vi "DG535.set internal trigger rate.vi"(0 "i ref in":refnum<vi>, 7 "internal trigger rate":dbl=0.001 min=0.001 max=1000000.0 format="%.3f", 11 "error in (no error)":errorcluster) -> (4 "i ref out":refnum<vi>, 15 "error out":errorcluster)   [LabVIEW 2014, in "DG535.lvlib"]
uses:
  DG535.lvlib
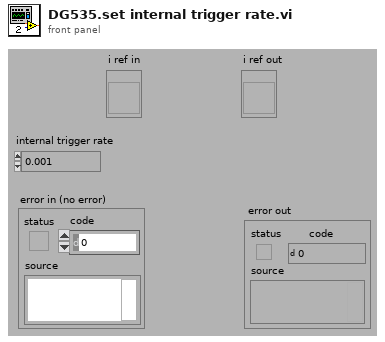
[diagram p1: front panel]
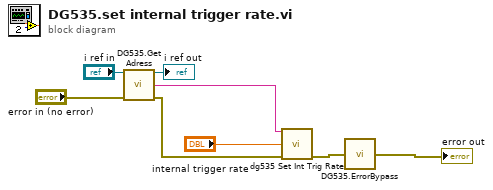
[diagram p0: block diagram]
diagram:
  n1 = call "DG535.Get Adress.vi"("i ref in"="i ref in", "error in (no error)"="error in (no error)") -> ("i ref out"=→"i ref out":refnum<vi>, "address"=w8:string, "error out"=w7:errorcluster)  [unwired: 10 in, 1 out]
  n2 = call "dg535 Set Int Trig Rate.vi"("address string"=w8, "internal trigger rate"="internal trigger rate", "error in"=w7) -> ("error out"=w5:errorcluster)  [unwired: 12 in]
  n3 = call "DG535.ErrorBypass.vi"("error in (no error)"=w5) -> ("error out"=→"error out":errorcluster)  [unwired: 14 in]
